vi "GetReadHead.vi"(8 "error in":errorcluster, 11 "camera.nit_c in":refnum<class "camera.lvclass">) -> (0 "error out":errorcluster, 2 "LastImageNumber":i64)   [LabVIEW 2020, in "camera.lvclass"]
uses:
  camera.lvclass
  camera.lvclass/camera.ctl
  lib/O-PL.dll
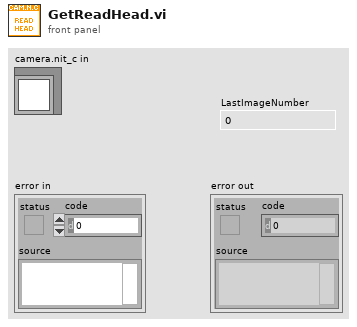
[diagram p1: front panel]
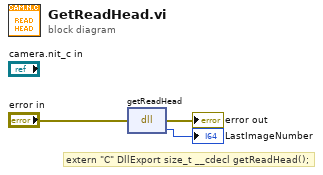
[diagram p0: block diagram]
diagram:
  # "extern \"C\" DllExport size_t __cdecl getReadHead();"
  n1 = dll-call lib="D:/UNSW - New/v0.8.3/lib/O-PL.dll" fn="getReadHead"(error in="error in") -> (error out=→"error out":errorcluster, "LastImageNumber"=→"LastImageNumber":i64)  [unwired: 2 in, 1 out]
